vi "RemoveBrackets.vi"(2 "String in":string) -> (6 "String out":string)   [LabVIEW 2020, in "Sgraph_lib_V1.lvlib"]
doc: "Andre Koelewijn, 2 jan 2021\n\nRemove all bracketed text from a string"
uses:
  Builds/Sgraph_lib_V1.lvlib
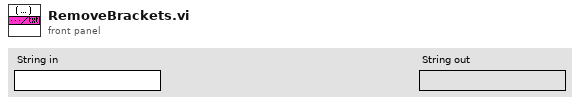
[diagram p1: front panel]
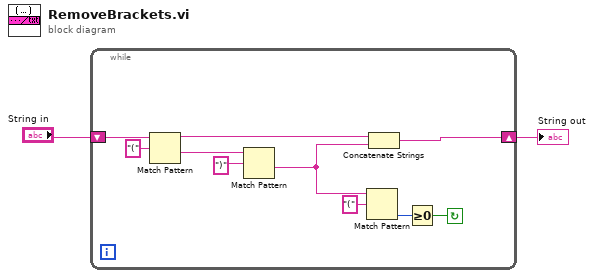
[diagram p0: block diagram]
diagram:
  n1 = while {
    shift-right: [w7] -> w1
    shift-left: "String in" -> [w12]
    stop <- w3 continue-if-true
    n2 = Match Pattern(string=w12, regular expression="(") -> (before substring=w8:string, after substring=w9:string)  [unwired: 1 in, 2 out]
    n3 = Match Pattern(string=w9, regular expression=")") -> (after substring=w5:string)  [unwired: 1 in, 3 out]
    n4 = Match Pattern(string=w5, regular expression="(") -> (offset past match=w4:i32)  [unwired: 1 in, 3 out]
    n5 = Concatenate Strings(w8, w5) -> (w7:string)
    n6 = Greater Or Equal To 0?(x=w4) -> (x >= 0?=w3:bool)
  }
  "String out" <- w1
